vi "BMU参数读取-Auto.vi"(7 "Socket":dbl, 8 "CAN端口":u16(ring), 9 "设备索引号":u16(ring), 10 "CAN卡类型":u32(ring)=21, 11 "从板号":u8=1) -> (3 "成功?":bool)   [LabVIEW 2013] (continued)
                  n842 = call <vilib>:"Close Config Data.vi"("error in (no error)"=w1345, "write file if changed (T)"=w1344, "refnum"=w1343) -> ("error out"=w1342:errorcluster, "file path"=w1339:path)  [unwired: 7 in]
                  n843 = call <vilib>:"MD5Checksum File.vi"("error in (no error)"=w1342, "Path"=w1339) -> ("error out"=w1340:errorcluster, "MD5 message-digest"=w1348:string)  [unwired: 8 in]
                  n844 = Equal?(x=w1348, y=w1347) -> (x = y?=w1346:bool)
                  n845 = Delete(path (use dialog)=w1339, error in=w1340) -> (error out=w1338:errorcluster)  [unwired: 3 in, 2 out]
                  n846 = call <vilib>:"Clear Errors.vi"("error in (no error)"=w1338) -> ()  [unwired: 6 in, 1 out]
                }
              }
              n847 = global write "配置文件全局.vi" "诊断标定读取地址"(w1318) -> ()
              n848 = And(x=w1319, y=w1320) -> (x .and. y?=w1321:bool)
              n849 = control-ref of="结果"() -> (w1326:refnum<vi>)
              n850 = case shown="真" w1321 {
                tunnel: w1307 -> [_ w1370]
                tunnel: w1326 -> [w1356 w1369]
                tunnel: w1320 -> [w1355 _]
                tunnel: w1319 -> [w1354 _]
                frame False {
                  n851 = stacked-sequence {
                    tunnel: w1354 -> [w1358 _]
                    tunnel: w1356 -> [w1357 w1364]
                    tunnel: w1355 -> [_ w1363]
                    frame #0 {
                      n852 = case shown="假" w1358 {
                        tunnel: w1357 -> [w1360 _]
                        frame False {
                          n853 = Build Array("文件格式错误") -> (w1361:string[])
                          n854 = call "表格编辑.vi"("新元素/子数组"=w1361, "活动单元格:单元格背景色"=u32 16711680, "MCListbox引用句柄"=w1360) -> ()  [unwired: 9 out]
                        }
                        frame True {
                        }
                      }
                    }
                    frame #1 {
                      n855 = case shown="假" w1363 {
                        tunnel: w1364 -> [w1366 _]
                        frame False {
                          n856 = Build Array("文件MD5码验证错误") -> (w1367:string[])
                          n857 = call "表格编辑.vi"("新元素/子数组"=w1367, "活动单元格:单元格背景色"=u32 16711680, "MCListbox引用句柄"=w1366) -> ()  [unwired: 9 out]
                        }
                        frame True {
                        }
                      }
                    }
                  }
                  n858 = call <vilib>:"Unset Busy.vi"() -> ()  [unwired: 11 in, 1 out]
                }
                frame True {
                  n859 = stacked-sequence {
                    seq-local: [w1375 _ _ _] -> [_ w1603 w1697 _]
                    seq-local: [w1373 _ _ _] -> [_ w1581 _ _]
                    tunnel: w1370 -> [w1371 _ _ _]
                    tunnel: w1369 -> [w1388 _ _ w1724]
                    frame #0 {
                      w1372 = string[][] []
                      w1385 = "总信息" ("section")
                      n860 = local write "路径"(w1371) -> ()
                      n861 = call <vilib>:"Open Config Data.vi"("create file if necessary (T)"=FALSE, "configuration file path"=w1371) -> ("error out"=w1376:errorcluster, "refnum"=w1375:T26)  [unwired: 7 in, 1 out]
                      n862 = call <vilib>:"Get Key Names.vi"("section"=w1385, "error in (no error)"=w1376, "refnum"=w1375) -> ("key names"=w1384:string[], "refnum out"=w1386:T26)  [unwired: 5 in, 2 out]
                      n863 = for {
                        tunnel: w1386 -> [w1392]
                        tunnel: w1385 -> [w1391]
                        tunnel: w1384 -> [w1390] mode=indexing
                        tunnel: [w1389] -> w1381 mode=indexing
                        n864 = call-poly <vilib>:"Read Key.vi"("section"=w1391, "key"=w1390, "refnum"=w1392) -> ("value"=w1389:string)  [unwired: 5 in, 3 out]
                      }
                      n865 = Index Array(array=w1381) -> (element #1=w1374:string, element #2=w1379:string)  [unwired: 2 in]
                      n866 = Decimal String To Number(string=w1374) -> (number=w1373:i32)  [unwired: 2 in, 1 out]
                      n867 = Concatenate Strings("正在读取" ("字符串"), w1379, "的配置文件" ("字符串")) -> (w1377:string)
                      n868 = Build Array(w1377) -> (w1382:string[])
                      n869 = call "表格编辑.vi"("新元素/子数组"=w1382, "活动单元格:单元格背景色"=u32 6618880, "MCListbox引用句柄"=w1388) -> ()  [unwired: 9 out]
                      n870 = local write "项目信息"(w1372) -> ()
                      n871 = local write "项目信息 2"(w1372) -> ()
                    }
                    frame #1 {
                      w1563 = 20 ("长度")
                      w1604 = "主板" ("section")
                      n872 = call <vilib>:"Get Key Names.vi"("section"=w1604, "refnum"=w1603) -> ("key names"=w1405:string[], "refnum out"=w1605:T26)  [unwired: 6 in, 2 out]
                      n873 = for {
                        tunnel: w1605 -> [w1617]
                        tunnel: w1604 -> [w1616]
                        tunnel: w1405 -> [w1615] mode=indexing
                        tunnel: [w1614] -> w1404 mode=indexing
                        n874 = call-poly <vilib>:"Read Key.vi"("section"=w1616, "key"=w1615, "refnum"=w1617) -> ("value"=w1614:string)  [unwired: 5 in, 3 out]
                      }
                      n875 = Search 1D Array(1D array=w1405, element="总电压过高一级" ("元素"), start index (0)=0 ("开始索引(0)")) -> (index of element=w1485:i32)
                      n876 = Search 1D Array(1D array=w1405, element="风机开启温度" ("元素"), start index (0)=w1485) -> (index of element=w1476:i32)
                      n877 = Search 1D Array(1D array=w1405, element="电池串联" ("元素"), start index (0)=w1476) -> (index of element=w1474:i32)
                      n878 = Decrement(x=w1485) -> (x-1=w1602:i32)
                      n879 = Array Subset(array=w1405, index=1 ("索引"), length=w1602) -> (w1450:string[])
                      n880 = Array Subset(array=w1404, index=1 ("索引"), length=w1602) -> (w1447:string[])
                      n881 = Delete From Array(array=w1447, length=7 ("长度"), index=0 ("索引")) -> (deleted portion=w1444:string[], array with subset deleted=w1394:string[])
                      n882 = Delete From Array(array=w1450, length=7 ("长度"), index=0 ("索引")) -> (array with subset deleted=w1403:string[])  [unwired: 1 out]
                      n883 = Search 1D Array(1D array=w1405, element="分流器型号" ("元素")) -> (index of element=w1408:i32)  [unwired: 1 in]
                      n884 = Index Array(array=w1404, index=0 ("索引")) -> (element=w1578:string)
                      n885 = Decimal String To Number(string=w1578) -> (number=w1395:i32)  [unwired: 2 in, 1 out]
                      n886 = Search 1D Array(1D array=w1403, element="主板电池节数" ("元素")) -> (index of element=w1569:i32)  [unwired: 1 in]
                      n887 = Search 1D Array(1D array=w1403, element="主板温度起始值" ("元素")) -> (index of element=w1566:i32)  [unwired: 1 in]
                      n888 = Search 1D Array(1D array=w1403, element="第一个保险通道" ("元素")) -> (index of element=w1565:i32)  [unwired: 1 in]
                      n889 = Search 1D Array(1D array=w1403, element="主板温度个数" ("元素")) -> (index of element=w1567:i32)  [unwired: 1 in]
                      n890 = Search 1D Array(1D array=w1403, element="主板电压起始值" ("元素")) -> (index of element=w1568:i32)  [unwired: 1 in]
                      n891 = Search 1D Array(1D array=w1403, element="第1通道电压个数" ("元素")) -> (index of element=w1564:i32)  [unwired: 1 in]
                      n892 = Index Array(array=w1404, index=w1408) -> (element=w1407:string)
                      n893 = for {
                        N: 4 -> [_]
                        tunnel: w1444 -> [w1613] mode=indexing
                        tunnel: [w1612] -> w1593 mode=indexing
                        n894 = Fract/Exp String To Number(string=w1613) -> (number=w1612:dbl)  [unwired: 3 in, 1 out]
                      }
                      n895 = Increment(x=w1395) -> (x+1=w1577:i32)
                      n896 = Increment(x=w1395) -> (x+1=w1562:i32)
                      n897 = Increment(x=w1395) -> (x+1=w1575:i32)
                      n898 = Increment(x=w1395) -> (x+1=w1576:i32)
                      n899 = global write "读配置文件全局.vi" "从板个数"(w1395) -> ()
                      n900 = local write "从板个数"(w1395) -> ()
                      n901 = Decimal String To Number(string=w1407) -> (number=w1406:i32)  [unwired: 2 in, 1 out]
                      n902 = Index Array(array=w1444, index #1=4 ("索引"), index #2=5 ("索引"), index #3=6 ("索引")) -> (element #1=w1584:string, element #2=w1583:string, element #3=w1582:string)
                      n903 = Index Array(array=w1593) -> (element #1=w1591:dbl, element #2=w1590:dbl, element #3=w1589:dbl, element #4=w1588:dbl)  [unwired: 4 in]
                      n904 = global write "EV05全局变量1.vi" "分流器型号"(w1406) -> ()
                      n905 = Array Subset(array=w1394, index=w1569, length=w1577) -> (w1561:string[])
                      n906 = Array Subset(array=w1394, index=w1568, length=w1576) -> (w1559:string[])
                      n907 = Array Subset(array=w1394, index=w1567, length=w1575) -> (w1558:string[])
                      n908 = Array Subset(array=w1394, index=w1566, length=w1562) -> (w1557:string[])
                      n909 = Array Subset(array=w1394, index=w1565, length=20 ("长度")) -> (w1556:string[])
                      n910 = Array Subset(array=w1394, index=w1564, length=w1563) -> (w1560:string[])
                      n911 = Multiply(x=w1395, y=2) -> (x*y=w1396:i32)
                      n912 = control-ref of="项目信息2"() -> (w1596:refnum<vi>)
                      n913 = Array Subset(array=w1394, index=0 ("索引"), length=w1396) -> (w1393:string[])
                      n914 = Insert Into Array(array=w1561, new element #1=w1560, new element #2=w1559, new element #3=w1558, new element #4=w1557, new element #5=w1556) -> ()  [unwired: 1 in, 1 out]
                      n915 = property class="Clust (严格)"(reference=w1596) -> (reference out=w1594:refnum<vi>, "Value"=w1595:T10)  [unwired: 1 in, 1 out]
                      n916 = Multiply(x=w1395, y=2) -> (x*y=w1400:i32)
                      n917 = Array Subset(array=w1403, index=w1569, length=w1562) -> (w1434:string[])
                      n918 = Array Subset(array=w1403, index=w1568, length=w1562) -> (w1432:string[])
                      n919 = Array Subset(array=w1403, index=w1567, length=w1562) -> (w1431:string[])
                      n920 = Array Subset(array=w1403, index=w1566) -> (w1430:string[])  [unwired: 1 in]
                      n921 = Array Subset(array=w1403, index=w1565, length=w1563) -> (w1429:string[])
                      n922 = Array Subset(array=w1403, index=w1564, length=w1563) -> (w1433:string[])
                      n923 = Array Subset(array=w1403, index=0 ("索引"), length=w1400) -> (w1399:string[])
                      n924 = global write "读配置文件全局.vi" "表格输入"(w1393) -> ()
                      n925 = Build Array(w1399, w1393) -> (w1555:string[][])
                      n926 = Bundle(cluster=w1595, "电池额定容量(A)"=w1591, "使用者"=w1581, "电池实际容量(A)"=w1590, "车架(牌)号"=w1583, "配置文件版本"=w1582, "SOH(%)"=w1588, "SOC(%)"=w1589, "产品编号"=w1584) -> (w1421:T10)  [unwired: 1 in]
                      n927 = Transpose 2D Array(2D array=w1555) -> (transposed array=w1422:string[][])
                      n928 = Multiply(x=w1395, y=4) -> (x*y=w1426:i32)
                      n929 = Insert Into Array(array=w1434, new element #1=w1433, new element #2=w1432, new element #3=w1431, new element #4=w1430, new element #5=w1429) -> (w1428:string[])  [unwired: 1 in]
                      n930 = Add(x=w1426, y=44) -> (x+y=w1424:i32)
                      n931 = local write "项目信息"(w1422) -> ()
                      n932 = property class="Clust (严格)"(reference=w1594, "Value"=w1421) -> ()  [unwired: 1 in, 2 out]
                      n933 = global write "读配置文件全局.vi" "项目信息"(w1421) -> ()
                      n934 = Array Subset(array=w1404, index=w1474, length=15 ("长度")) -> (w1412:string[])
                      n935 = Array Subset(array=w1428, index=0 ("索引"), length=w1424) -> ()  [unwired: 1 out]
                      n936 = Array Subset(array=w1404, index=w1476, length=15 ("长度")) -> (w1481:string[])
                      n937 = Delete From Array(array=w1412, length=4 ("长度"), index=6 ("索引")) -> (deleted portion=w1468:string[], array with subset deleted=w1467:string[])
                      n938 = for {
                        tunnel: w1481 -> [w1609] mode=indexing
                        tunnel: [w1608] -> w1480 mode=indexing
                        n939 = Fract/Exp String To Number(string=w1609) -> (number=w1608:dbl)  [unwired: 3 in, 1 out]
                      }
                      n940 = for {
                        tunnel: w1467 -> [w1607] mode=indexing
                        tunnel: [w1606] -> w1466 mode=indexing
                        n941 = Fract/Exp String To Number(string=w1607) -> (number=w1606:dbl)  [unwired: 3 in, 1 out]
                      }
                      n942 = Array Subset(array=w1404, index=w1485, length=51 ("长度")) -> (w1554:string[])
                      n943 = for {
                        tunnel: w1554 -> [w1611] mode=indexing
                        tunnel: [w1610] -> w1553 mode=indexing
                        n944 = Fract/Exp String To Number(string=w1611) -> (number=w1610:dbl)  [unwired: 3 in, 1 out]
                      }
                      n945 = Index Array(array=w1466) -> (element #1=w1461:dbl, element #2=w1460:dbl, element #3=w1459:dbl, element #4=w1458:dbl, element #5=w1457:dbl, element #6=w1456:dbl, element #7=w1455:dbl, element #8=w1454:dbl, element #9=w1453:dbl, element #10=w1452:dbl, element #11=w1451:dbl)  [unwired: 11 in]
                      n946 = Delete From Array(array=w1480, length=7 ("长度"), index=0 ("索引")) -> (deleted portion=w1417:dbl[], array with subset deleted=w1478:dbl[])
                      n947 = Delete From Array(array=w1553, length=17 ("长度"), index=0 ("索引")) -> (deleted portion=w1414:dbl[], array with subset deleted=w1550:dbl[])
                      n948 = Array To Cluster(array=w1417) -> (cluster=w1479:T27)
                      n949 = global write "读配置文件全局.vi" "加热控制参数"(w1417) -> ()
                      n950 = Index Array(array=w1478) -> (element #1=w1442:dbl, element #2=w1441:dbl, element #3=w1440:dbl, element #4=w1439:dbl, element #5=w1438:dbl, element #6=w1437:dbl, element #7=w1436:dbl, element #8=w1435:dbl)  [unwired: 8 in]
                      n951 = Delete From Array(array=w1550, length=17 ("长度"), index=0 ("索引")) -> (deleted portion=w1413:dbl[], array with subset deleted=w1410:dbl[])
                      n952 = Index Array(array=w1468) -> (element #1=w1465:string, element #2=w1464:string, element #3=w1462:string, element #4=w1463:string)  [unwired: 4 in]
                      n953 = local write "加热控制参数"(w1479) -> ()
                      n954 = global write "读配置文件全局.vi" "一级故障"(w1414) -> ()
                      n955 = local read "一级故障 5"() -> (w1443:T13)
                      n956 = control-ref of="电池信息"() -> (w1472:refnum<vi>)
                      n957 = global write "读配置文件全局.vi" "二级故障"(w1413) -> ()
                      n958 = global write "读配置文件全局.vi" "三级故障"(w1410) -> ()
                      n959 = Bundle(cluster=w1443, "最大允许单体电压"=w1442, "最大允许总电压"=w1438, "最小允许单体电压"=w1441, "最大允许充电电流"=w1440, "最小允许充电电流"=w1439, "最大允许充电温度"=w1437, "最小允许充电温度"=w1436, "电流步长"=w1435) -> (w1416:T13)
                      n960 = property class="Clust (严格)"(reference=w1472) -> (reference out=w1473:refnum<vi>, "Value"=w1471:T14)  [unwired: 1 in, 1 out]
                      n961 = Bundle(cluster=w1471, "电池串联"=w1461, "电池并联"=w1460, "累计放电总安时"=w1454, "电池包额定容量"=w1459, "电池包额定能量(kWh)"=w1458, "电池包额定总电压"=w1457, "累计充电总安时"=w1455, "电池充满次数"=w1452, "电池放空次数"=w1453, "电池充电次数"=w1451, "电池生产日期"=w1462, "电池厂家"=w1465, "电池类型"=w1464, "电池包组号"=w1463, "实际容量"=w1456) -> (w1411:T14)  [unwired: 2 in]
                      n962 = Cluster To Array(cluster=w1416) -> (array=w1415:dbl[])
                      n963 = local write "一级故障 5"(w1416) -> ()
                      n964 = global write "读配置文件全局.vi" "充电控制参数"(w1415) -> ()
                      n965 = Index Array(array=w1414) -> (element #1=w1543:dbl, element #2=w1542:dbl, element #3=w1541:dbl, element #4=w1540:dbl, element #5=w1539:dbl, element #6=w1538:dbl, element #7=w1537:dbl, element #8=w1536:dbl, element #9=w1535:dbl, element #10=w1534:dbl, element #11=w1533:dbl, element #12=w1532:dbl, element #13=w1531:dbl, element #14=w1530:dbl, element #15=w1529:dbl, element #16=w1528:dbl, element #17=w1527:dbl)  [unwired: 17 in]
                      n966 = global write "读配置文件全局.vi" "电池信息"(w1411) -> ()
                      n967 = Index Array(array=w1413) -> (element #1=w1510:dbl, element #2=w1511:dbl, element #3=w1512:dbl, element #4=w1513:dbl, element #5=w1514:dbl, element #6=w1515:dbl, element #7=w1516:dbl, element #8=w1517:dbl, element #9=w1518:dbl, element #10=w1519:dbl, element #11=w1520:dbl, element #12=w1521:dbl, element #13=w1522:dbl, element #14=w1523:dbl, element #15=w1524:dbl, element #16=w1525:dbl, element #17=w1526:dbl)  [unwired: 17 in]
                      n968 = Index Array(array=w1410) -> (element #1=w1505:dbl, element #2=w1504:dbl, element #3=w1503:dbl, element #4=w1502:dbl, element #5=w1501:dbl, element #6=w1500:dbl, element #7=w1499:dbl, element #8=w1498:dbl, element #9=w1497:dbl, element #10=w1496:dbl, element #11=w1495:dbl, element #12=w1494:dbl, element #13=w1493:dbl, element #14=w1492:dbl, element #15=w1491:dbl, element #16=w1490:dbl, element #17=w1489:dbl)  [unwired: 17 in]
                      n969 = control-ref of="一级故障 3"() -> (w1488:refnum<vi>)
                      n970 = control-ref of="一级故障 2"() -> (w1507:refnum<vi>)
                      n971 = property class="Clust (严格)"(reference=w1507) -> (reference out=w1509:refnum<vi>, "Value"=w1508:T11)  [unwired: 1 in, 1 out]
                      n972 = property class="Clust (严格)"(reference=w1488) -> (reference out=w1487:refnum<vi>, "Value"=w1506:T11)  [unwired: 1 in, 1 out]
                      n973 = property class="Clust (严格)"(reference=w1473, "Value"=w1411) -> ()  [unwired: 1 in, 2 out]
                      n974 = Bundle(cluster=w1508, "总电压过高"=w1510, "整组电压不均衡"=w1514, "SOC过高"=w1522, "单体电压过高"=w1518, "总电压过低"=w1511, "温度过高"=w1512, "温度过低"=w1513, "单组电压不均衡"=w1515, "整组温度不均衡"=w1516, "单组温度不均衡"=w1517, "单体电压过低"=w1519, "充电电流过高"=w1520, "放电电流过高"=w1521, "SOC过低"=w1523, "内阻过大"=w1524, "极柱温度过高"=w1525, "SOH过低"=w1526) -> (w1419:T11)
                      n975 = property class="Clust (严格)"(reference=w1509, "Value"=w1419) -> ()  [unwired: 1 in, 2 out]
                      n976 = Bundle(cluster=w1506, "总电压过高"=w1505, "整组电压不均衡"=w1501, "SOC过高"=w1493, "单体电压过高"=w1497, "总电压过低"=w1504, "温度过高"=w1503, "温度过低"=w1502, "单组电压不均衡"=w1500, "整组温度不均衡"=w1499, "单组温度不均衡"=w1498, "单体电压过低"=w1496, "充电电流过高"=w1495, "放电电流过高"=w1494, "SOC过低"=w1492, "内阻过大"=w1491, "极柱温度过高"=w1490, "SOH过低"=w1489) -> (w1418:T11)
                      n977 = property class="Clust (严格)"(reference=w1487, "Value"=w1418) -> ()  [unwired: 1 in, 2 out]
                      n978 = control-ref of="一级故障"() -> (w1546:refnum<vi>)
                      n979 = property class="Clust (严格)"(reference=w1546) -> (reference out=w1544:refnum<vi>, "Value"=w1545:T11)  [unwired: 1 in, 1 out]
                      n980 = Bundle(cluster=w1545, "总电压过高"=w1543, "整组电压不均衡"=w1539, "SOC过高"=w1531, "单体电压过高"=w1535, "总电压过低"=w1542, "温度过高"=w1541, "温度过低"=w1540, "单组电压不均衡"=w1538, "整组温度不均衡"=w1537, "单组温度不均衡"=w1536, "单体电压过低"=w1534, "充电电流过高"=w1533, "放电电流过高"=w1532, "SOC过低"=w1530, "内阻过大"=w1529, "极柱温度过高"=w1528, "SOH过低"=w1527) -> (w1420:T11)
                      n981 = property class="Clust (严格)"(reference=w1544, "Value"=w1420) -> ()  [unwired: 1 in, 2 out]
                    }
                    frame #2 {
                      w1682 = 1 ("索引")
                      # "均衡计算-电压高阀值1级"
                      n982 = call <vilib>:"Get Section Names.vi"("refnum"=w1697) -> ("section names"=w1698:string[], "refnum out"=w1702:T26)  [unwired: 8 in, 1 out]
                      n983 = local read "从板号"() -> (w1680:u8)
                      n984 = Delete From Array(array=w1698, length=2 ("长度"), index=0 ("索引")) -> (array with subset deleted=w1701:string[])  [unwired: 1 out]
                      n985 = for {
                        tunnel: w1701 -> [w1718] mode=indexing
                        tunnel: w1702 -> [w1719]
                        tunnel: [w1711] -> w1679 mode=indexing
                        tunnel: [w1710] -> w1623
                        n986 = call <vilib>:"Get Key Names.vi"("section"=w1718, "refnum"=w1719) -> ("key names"=w1710:string[], "refnum out"=w1717:T26)  [unwired: 6 in, 2 out]
                        n987 = for {
                          tunnel: w1710 -> [w1723] mode=indexing
                          tunnel: w1718 -> [w1722]
                          tunnel: w1717 -> [w1721]
                          tunnel: [w1720] -> w1711 mode=indexing
                          n988 = call-poly <vilib>:"Read Key.vi"("section"=w1722, "key"=w1723, "refnum"=w1721) -> ("value"=w1720:string)  [unwired: 5 in, 3 out]
                        }
                        n989 = Index Array(array=w1711, index=0 ("索引")) -> (element=w1714:string)
                        n990 = local read "输出数组"() -> (w1715:string[][])
                        n991 = Decimal String To Number(string=w1714) -> (number=w1713:i32)  [unwired: 2 in, 1 out]
                        n992 = Decrement(x=w1713) -> (x-1=w1709:i32)
                        n993 = Replace Array Subset(array=w1715, new element=w1711, index (col)=w1709) -> (w1712:string[][])  [unwired: 1 in]
                        n994 = local write "输出数组"(w1712) -> ()
                      }
                      "key names" <- w1623
                      n995 = Decrement(x=w1680) -> (x-1=w1696:u8)
                      n996 = Index Array(array=w1679, index (row)=w1696) -> (element=w1622:string[])  [unwired: 1 in]
                      n997 = Search 1D Array(1D array=w1623, element="风机开启温度" ("元素")) -> (index of element=w1685:i32)  [unwired: 1 in]
                      n998 = Search 1D Array(1D array=w1623, element="电压过高一级" ("元素"), start index (0)=w1685) -> (index of element=w1648:i32)
                      n999 = Search 1D Array(1D array=w1623, element="均衡计算-电压高阀值1级" ("元素"), start index (0)=w1648) -> (index of element=w1646:i32)
                      n1000 = Array Subset(array=w1622, index=w1646, length=17 ("长度")) -> (w1645:string[])
                      n1001 = Decrement(x=w1685) -> (x-1=w1683:i32)
                      n1002 = Array Subset(array=w1622, index=w1682, length=w1683) -> (w1620:string[])
                      n1003 = Array Subset(array=w1622, index=w1648, length=21 ("长度")) -> (w1694:string[])
                      n1004 = Array Subset(array=w1623, index=w1682, length=w1683) -> (w1659:string[])
                      n1005 = Index Array(array=w1622, index=0 ("索引")) -> (element=w1654:string)
                      n1006 = Array Subset(array=w1622, index=w1685, length=7 ("长度")) -> (w1688:string[])
                      n1007 = for {
                        tunnel: w1645 -> [w1704] mode=indexing
                        tunnel: [w1703] -> w1644 mode=indexing
                        n1008 = Fract/Exp String To Number(string=w1704) -> (number=w1703:dbl)  [unwired: 3 in, 1 out]
                      }
                      n1009 = for {
                        tunnel: w1694 -> [w1706] mode=indexing
                        tunnel: [w1705] -> w1695 mode=indexing
                        n1010 = Fract/Exp String To Number(string=w1706) -> (number=w1705:dbl)  [unwired: 3 in, 1 out]
                      }
                      n1011 = Decimal String To Number(string=w1654) -> (number=w1653:i32)  [unwired: 2 in, 1 out]
                      n1012 = for {
                        tunnel: w1688 -> [w1708] mode=indexing
                        tunnel: [w1707] -> w1656 mode=indexing
                        n1013 = Fract/Exp String To Number(string=w1708) -> (number=w1707:dbl)  [unwired: 3 in, 1 out]
                      }
                      n1014 = global write "读配置文件全局2.vi" "从板板号"(w1653) -> ()
                      n1015 = Delete From Array(array=w1695, length=7 ("长度"), index=0 ("索引")) -> (deleted portion=w1658:dbl[], array with subset deleted=w1691:dbl[])
                      n1016 = Array To Cluster(array=w1656) -> (cluster=w1678:T27)
                      n1017 = Delete From Array(array=w1691, length=7 ("长度"), index=0 ("索引")) -> (deleted portion=w1651:dbl[], array with subset deleted=w1652:dbl[])
                      n1018 = local write "加热控制参数"(w1678) -> ()
                      n1019 = global write "读配置文件全局2.vi" "加热控制参数"(w1656) -> ()
                      n1020 = Array To Cluster(array=w1658) -> (cluster=w1662:T27)
                      n1021 = Array To Cluster(array=w1652) -> (cluster=w1660:T27)
                      n1022 = Array To Cluster(array=w1651) -> (cluster=w1661:T27)
                      n1023 = global write "读配置文件全局2.vi" "三级故障阀值"(w1652) -> ()
                      n1024 = global write "读配置文件全局2.vi" "一级故障阀值"(w1658) -> ()
                      n1025 = global write "读配置文件全局2.vi" "二级故障阀值"(w1651) -> ()
                      n1026 = local write "一级故障 6"(w1662) -> ()
                      n1027 = local write "一级故障 8"(w1660) -> ()
                      n1028 = local write "一级故障 7"(w1661) -> ()
                      n1029 = Search 1D Array(1D array=w1659, element="第1通道电压个数" ("元素")) -> (index of element=w1670:i32)  [unwired: 1 in]
                      n1030 = Search 1D Array(1D array=w1659, element="电压个数" ("元素")) -> ()  [unwired: 1 in, 1 out]
                      n1031 = Search 1D Array(1D array=w1659, element="温度个数" ("元素")) -> (index of element=w1672:i32)  [unwired: 1 in]
                      n1032 = Search 1D Array(1D array=w1659, element="第一个保险通道" ("元素")) -> (index of element=w1671:i32)  [unwired: 1 in]
                      n1033 = Array Subset(array=w1620, length=2 ("长度")) -> (w1667:string[])  [unwired: 1 in]
                      n1034 = Array Subset(array=w1620, index=w1672, length=2 ("长度")) -> (w1665:string[])
                      n1035 = Array Subset(array=w1620, index=w1671, length=20 ("长度")) -> (w1664:string[])
                      n1036 = Array Subset(array=w1620, index=w1670, length=20 ("长度")) -> (w1666:string[])
                      n1037 = Array Subset(array=w1620, length=27 ("长度")) -> (w1619:string[])  [unwired: 1 in]
                      n1038 = Insert Into Array(array=w1667, new element #1=w1666, new element #2=w1665, new element #3=w1664) -> ()  [unwired: 1 in, 1 out]
                      n1039 = Build Array(string[] ["电压个数", "温度个数", "第一个保险通道", "第一个保险位置", "第二个保险通道", "第二个保险位置", "第三个保险通道", "第三个保险位置", "第四个保险通道", "第四个保险位置", "第五个保险通道", "第五个保险位置", "第六个保险通道", "第六个保险位置", "第七个保险通道", "第七个保险位置", "第八个保险通道", "第八个保险位置", "第九个保险通道", "第九个保险位置", "第十个保险通道", "第十个保险位置", "第1通道电压个数", "第2通道电压个数", "第3通道电压个数", "第4通道电压个数", "第5通道电压个数"], w1619) -> (w1663:string[][])
                      n1040 = global write "读配置文件全局2.vi" "表格"(w1619) -> ()
                      n1041 = Index Array(array=w1644) -> (element #1=w1641:dbl, element #2=w1640:dbl, element #3=w1639:dbl, element #4=w1638:dbl, element #5=w1637:dbl, element #6=w1636:dbl, element #7=w1635:dbl, element #8=w1634:dbl, element #9=w1633:dbl, element #10=w1632:dbl, element #11=w1631:dbl, element #12=w1630:dbl, element #13=w1629:dbl, element #14=w1628:dbl, element #15=w1627:dbl, element #16=w1626:dbl, element #17=w1625:dbl, element #18=w1624:dbl)  [unwired: 18 in]
                      n1042 = Transpose 2D Array(2D array=w1663) -> (transposed array=w1657:string[][])
                      n1043 = local write "项目信息 2"(w1657) -> ()
                      n1044 = local read "均衡参数"() -> (w1643:T18)
                      n1045 = Bundle(cluster=w1643, "充电结束电压(90%)"=w1634, "充电结束电压(91%)"=w1633, "充电结束电压(92%)"=w1632, "充电结束电压(93%)"=w1631, "充电结束电压(94%)"=w1630, "均衡计算-电压高阀值1级"=w1641, "均衡计算-电压高阀值2级"=w1640, "均衡计算-电压低阀值1级"=w1639, "均衡计算-电压低阀值2级"=w1638, "均衡计算-最低电压阀值"=w1637, "均衡停止-最低电压阀值"=w1636, "均衡计算-电压极差阀值"=w1635, "充电结束电压(95%)"=w1629, "充电结束电压(96%)"=w1628, "充电结束电压(97%)"=w1627, "充电结束电压(98%)"=w1626, "充电结束电压(99%)"=w1625, "充电结束电压(100%)"=w1624) -> (w1642:T18)
                      n1046 = local write "均衡参数"(w1642) -> ()
                    }
                    frame #3 {
                      n1047 = call <vilib>:"Unset Busy.vi"() -> ()  [unwired: 11 in, 1 out]
                      n1048 = Build Array("读取完成") -> (w1727:string[])
                      n1049 = property on="全部写入" class="Bool (严格)"("DisabledEnum"=0) -> ()  [unwired: 2 in, 2 out]
                      n1050 = call "表格编辑.vi"("新元素/子数组"=w1727, "活动单元格:单元格背景色"=u32 6618880, "MCListbox引用句柄"=w1724) -> ()  [unwired: 9 out]
                    }
                  }
                }
              }
            }
            frame #2 {
              (unwired) "均衡参数"
              # "去掉加热控制信息 20140106"
              n1051 = local read "主从选择"() -> (w1732:enum32{"主板", "从板"})
              n1052 = case shown="\"主板\", 默认" w1732 {
                tunnel: [string[] ["项目信息", "一级故障阀值", "二级故障阀值", "三级故障阀值", "加热控制信息", "充电控制信息", "电池信息", "二维码"] string[] ["从板信息", "一级故障阀值", "二级故障阀值", "三级故障阀值", "二维码"]] -> w1731
                frame "主板", Default {
                }
                frame "从板" {
                }
              }
              n1053 = Array Size(array=w1731) -> (size(s)=w1730:i32)
              n1054 = for {
                tunnel: w1731 -> [w1748] mode=indexing
                tunnel: w1732 -> [w1736]
                tunnel: w1730 -> [w1740]
                tunnel: [w1735] -> w1729
                i -> [w1737]
                n1055 = case shown="\"主板\", 默认" w1736 {
                  tunnel: [w2045 w2076] -> w1742
                  tunnel: [w2044 w2077] -> w1743
                  tunnel: w1748 -> [w2041 w2073]
                  tunnel: [u8 0 ("板号") w2074] -> w1747
                  tunnel: [u8 0 ("板号") u8 0 ("板号")] -> w1746
                  tunnel: [w2040 w2072] -> w1744
                  frame "主板", Default {
                    n1056 = case shown="\"项目信息\"" w2041 {
                      tunnel: [_ u8[] [1, 2, 3, 4, 5, 6, 13, 8, 7, 9, 10, 11, 12] u8[] [1] u8[] [1] u8[] [2] u8[] [3] u8[] [1] u8[] [2] u8[] [1, 2, 3] u8[] [1, 2, 3, 4]] -> w2045
                      tunnel: [_ u8 128 ("命令") u8 140 ("命令") u8 129 ("命令") u8 129 ("命令") u8 129 ("命令") u8 130 ("命令") u8 130 ("命令") u8 131 ("命令") u8 132 ("命令")] -> w2044
                      tunnel: [_ string[] ["产品编号", "电压个数", "通道电压数", "电压起始值", "温度个数", "温度起始值", "保险位置", "电池额定实际容量", "SOC", "配置文件版本", "参数修改记录", "车牌号", "SOH"] string[] ["读二维码"] string[] ["一级故障阀值"] string[] ["二级故障阀值"] string[] ["三级故障阀值"] string[] ["加热控制参数"] string[] ["充电控制参数"] _ string[] ["电池信息1", "电池包组号", "充放电安时", "电池充放电次数"]] -> w2040
                      frame "假", Default {
                      }
                      frame "项目信息" {
                      }
                      frame "二维码" {
                      }
                      frame "一级故障阀值" {
                      }
                      frame "二级故障阀值" {
                      }
                      frame "三级故障阀值" {
                      }
                      frame "加热控制信息" {
                      }
                      frame "充电控制信息" {
                      }
                      frame "历史信息" {
                      }
                      frame "电池信息" {
                      }
                    }
                  }
                  frame "从板" {
                    n1057 = case shown="\"二维码\"" w2073 {
                      tunnel: [_ u8 0 ("命令") u8 10 ("命令") u8 2 ("命令") u8 2 ("命令") u8 2 ("命令") u8 3 ("命令") u8 6 ("命令")] -> w2077
                      tunnel: [_ u8[] [6, 1, 2, 3, 4, 5] u8[] [1] u8[] [1] u8[] [2] u8[] [3] u8[] [1, 2, 3, 4, 5, 6, 7] u8[] [1, 2]] -> w2076
                      tunnel: [_ string[] ["从板号", "电压起始值", "通道电压节数", "保险位置", "温度起始值", "加热控制参数"] string[] ["读二维码"] string[] ["一级故障阀值"] string[] ["二级故障阀值"] string[] ["三级故障阀值"] string[] ["电池包信息1", "电池包序号", "充放电安时", "充电次数时间", "SOC", "车牌号", "充电参数"] string[] ["均衡阀值", "充电结束电压"]] -> w2072
                      frame "假", Default {
                      }
                      frame "从板信息" {
                      }
                      frame "二维码" {
                      }
                      frame "一级故障阀值" {
                      }
                      frame "二级故障阀值" {
                      }
                      frame "三级故障阀值" {
                      }
                      frame "快换参数" {
                      }
                      frame "均衡参数" {
                      }
                    }
                    n1058 = local read "从板号"() -> (w2074:u8)
                  }
                }
                n1059 = Increment(x=w1737) -> (x+1=w1739:i32)
                n1060 = Equal?(x=w1740, y=w1739) -> (x = y?=w1738:bool)
                n1061 = case shown="\"从板\"" w1736 {
                  tunnel: w1737 -> [w2011 w2025]
                  frame "主板", Default {
                    n1062 = case shown="0, 默认" w2011 {
                      tunnel: [T9."项目信息" ("主从板") T9."一级故障阀值" ("主从板") T9."二级故障阀值" ("主从板") T9."三级故障阀值" ("主从板") T9."控制参数" ("主从板") T9."电池信息" ("主从板")] -> w2010
                      frame 0, Default {
                        n1063 = local write "1"(TRUE ("1")) -> ()
                      }
                      frame 1 {
                        n1064 = local write "1 2"(TRUE ("1 2")) -> ()
                      }
                      frame 2 {
                        n1065 = local write "1 3"(TRUE ("1 3")) -> ()
                      }
                      frame 3 {
                        n1066 = local write "1 4"(TRUE ("1 4")) -> ()
                      }
                      frame 4, 5 {
                        n1067 = local write "1 5"(TRUE ("1 5")) -> ()
                      }
                      frame 6 {
                        n1068 = local write "1 11"(TRUE ("1 11")) -> ()
                      }
                    }
                    n1069 = local write "主板2"(w2010) -> ()
                  }
                  frame "从板" {
                    n1070 = case shown="4" w2025 {
                      tunnel: [T20."从板信息" ("等级 2") T20."从板信息" ("等级 2") T20."一级故障阀值" ("等级 2") T20."二级故障阀值" ("等级 2") T20."三级故障阀值" ("等级 2") T20."快换参数" ("等级 2") T15."从板信息" ("等级 2")] -> w2024
                      frame 99, Default {
                        n1071 = local write "1 6"(TRUE ("1 6")) -> ()
                      }
                      frame 0 {
                        n1072 = local write "1 6"(TRUE ("1 6")) -> ()
                      }
                      frame 1 {
                        n1073 = local write "1 7"(TRUE ("1 7")) -> ()
                      }
                      frame 2 {
                        n1074 = local write "1 8"(TRUE ("1 8")) -> ()
                      }
                      frame 3 {
                        n1075 = local write "1 9"(TRUE ("1 9")) -> ()
                      }
                      frame 5 {
                        n1076 = local write "1 10"(TRUE ("1 10")) -> ()
                      }
                      frame 4 {
                        n1077 = local write "1 12"(TRUE ("1 10")) -> ()
                      }
                    }
                    n1078 = local write "等级 2"(w2024) -> ()
                  }
                }
                n1079 = Array Size(array=w1742) -> (size(s)=w1741:i32)
                n1080 = local write "命令"(w1743) -> ()
                n1081 = Build Array(w1746) -> (w1745:u8[])
                n1082 = while {
                  tunnel: w1743 -> [w1780]
                  tunnel: w1747 -> [w1779]
                  tunnel: w1745 -> [w1778]
                  tunnel: w1741 -> [w1774]
                  tunnel: w1738 -> [w1777]
                  tunnel: w1736 -> [w1771]
                  tunnel: [w1770] -> w1735
                  shift-right: [w1769] -> _
                  shift-left: w1744 -> [w1750]
                  shift-right: [w1760] -> _
                  shift-left: w1742 -> [w1749]
                  i -> [w1775]
                  stop <- w1770 stop-if-true
                  n1083 = local read "强制终止读写标记"() -> (w1766:bool)
                  n1084 = Array Size(array=w1750) -> (size(s)=w1768:i32)
                  n1085 = Increment(x=w1775) -> (x+1=w1776:i32)
                  n1086 = Greater Than 0?(x=w1768) -> (x > 0?=w1767:bool)
                  n1087 = Equal?(x=w1774, y=w1776) -> (x = y?=w1772:bool)
                  n1088 = Not(x=w1766) -> (.not. x?=w1765:bool)
                  n1089 = And(x=w1765, y=w1767) -> (x .and. y?=w1764:bool)
                  n1090 = Delete From Array(array=w1750, length=1 ("长度"), index=0 ("索引")) -> (deleted portion=w1756:string[], array with subset deleted=w1761:string[])
                  n1091 = Index Array(array=w1756, index=0 ("索引")) -> (element=w1754:string)
                  n1092 = Delete From Array(array=w1749, length=1 ("长度"), index=0 ("索引")) -> (deleted portion=w1752:u8[], array with subset deleted=w1757:u8[])
                  n1093 = Index Array(array=w1752, index=0 ("索引")) -> (element=w1751:u8)
                  n1094 = case shown="真" w1764 {
                    tunnel: w1780 -> [_ w1796]
                    tunnel: w1751 -> [_ w1795]
                    tunnel: w1779 -> [_ w1794]
                    tunnel: w1778 -> [_ w1793]
                    tunnel: w1754 -> [_ w1792]
                    tunnel: w1777 -> [_ w1791]
                    tunnel: w1772 -> [_ w1790]
                    tunnel: w1771 -> [_ w1789]
                    tunnel: [string[] [] w1785] -> w1769
                    tunnel: w1761 -> [_ w1788]
                    tunnel: [u8[] [] w1783] -> w1760
                    tunnel: w1757 -> [_ w1787]
                    tunnel: w1750 -> [_ w1786]
                    tunnel: w1749 -> [_ w1784]
                    frame False {
                    }
                    frame True {
                      n1095 = while {
                        tunnel: w1796 -> [w1812]
                        tunnel: w1795 -> [w1811]
                        tunnel: w1794 -> [w1810]
                        tunnel: w1793 -> [w1809]
                        tunnel: w1792 -> [w1807]
                        tunnel: w1791 -> [w1806]
                        tunnel: w1790 -> [w1805]
                        tunnel: w1789 -> [w1804]
                        tunnel: w1788 -> [w1800]
                        tunnel: w1787 -> [w1798]
                        tunnel: w1786 -> [w1801]
                        tunnel: [w1802] -> w1785
                        tunnel: w1784 -> [w1799]
                        tunnel: [w1797] -> w1783
                        i -> [w1803]
                        stop <- w1808 stop-if-true
                        n1096 = stacked-sequence {
                          seq-local: [_ _ _ _ w1960 _ _] -> [_ _ _ _ _ w1976 _]
                          tunnel: w1812 -> [_ _ _ w1951 _ _ _]
                          tunnel: w1811 -> [_ _ _ w1950 _ _ _]
                          tunnel: w1810 -> [_ _ _ w1949 _ _ _]
                          tunnel: w1809 -> [_ _ _ w1948 _ _ _]
                          tunnel: [_ _ _ _ w1961 _ _] -> w1808
                          tunnel: w1807 -> [w1814 _ _ _ _ w1975 _]
                          tunnel: w1806 -> [_ _ _ _ _ _ w2003]
                          tunnel: w1805 -> [_ _ _ _ _ _ w2001]
                          tunnel: w1804 -> [w1813 _ _ _ _ _ _]
                          tunnel: w1803 -> [_ _ _ _ _ _ _]
                          tunnel: [_ _ _ _ _ w1974 _] -> w1802
                          tunnel: w1801 -> [_ _ _ _ _ w1973 _]
                          tunnel: w1800 -> [_ _ _ _ _ w1972 _]
                          tunnel: w1799 -> [_ _ _ _ _ w1971 _]
                          tunnel: w1798 -> [_ _ _ _ _ w1970 _]
                          tunnel: [_ _ _ _ _ w1969 _] -> w1797
                          frame #0 {
                            n1097 = case shown="\"从板\"" w1813 {
                              tunnel: w1814 -> [w1815 w1906]
                              frame "主板", Default {
                                n1098 = case shown="\"电压个数\"" w1815 {
                                frame "假", Default {
                                }
                                frame "产品编号" {
                                n1099 = control-ref of="产品编号"() -> (w1817:refnum<vi>)
                                n1100 = property class="Str"(reference=w1817, "Value"="") -> ()  [unwired: 1 in, 2 out]
                                }
                                frame "电压个数" {
                                n1101 = local read "从板个数"() -> (w1818:dbl)
                                n1102 = control-ref of="项目信息"() -> (w1822:refnum<vi>)
                                n1103 = for {
                                N: w1818 -> [_]
                                tunnel: [""] -> w1821 mode=indexing
                                }
                                n1104 = call "表格数据输入-8.6.vi"("行数"=u32 0, "列数"=u32 1, "字符串数组"=w1821, "表格引用"=w1822) -> ()  [unwired: 8 in]
                                }
                                frame "通道电压数" {
                                n1105 = disable-structure shown="禁用" {
                                frame Disabled {
                                n1106 = control-ref of="项目信息"() -> (w1828:refnum<vi>)
                                n1107 = for {
                                N: 20 -> [_]
                                tunnel: [""] -> w1827 mode=indexing
                                }
                                n1108 = local read "从板个数"() -> (w1829:dbl)
                                n1109 = Increment(x=w1829) -> (x+1=w1825:dbl)
                                n1110 = call "表格数据输入-8.6.vi"("行数"=w1825, "列数"=u32 1, "字符串数组"=w1827, "表格引用"=w1828) -> ()  [unwired: 8 in]
                                }
                                frame Enabled {
                                }
                                }
                                }
                                frame "电压起始值" {
                                n1111 = disable-structure shown="禁用" {
                                frame Disabled {
                                n1112 = local read "从板个数"() -> (w1833:dbl)
                                n1113 = Increment(x=w1833) -> (x+1=w1832:dbl)
                                n1114 = control-ref of="项目信息"() -> (w1839:refnum<vi>)
                                n1115 = for {
                                N: w1832 -> [_]
                                tunnel: [""] -> w1838 mode=indexing
                                }
                                n1116 = Multiply(x=u8 1, y=w1833) -> (x*y=w1835:dbl)
                                n1117 = Add(x=w1835, y=u8 21) -> (x+y=w1831:dbl)
                                n1118 = call "表格数据输入-8.6.vi"("行数"=w1831, "列数"=u32 1, "字符串数组"=w1838, "表格引用"=w1839) -> ()  [unwired: 8 in]
                                }
                                frame Enabled {
                                }
                                }
                                }
                                frame "温度个数" {
                                n1119 = local read "从板个数"() -> (w1843:dbl)
                                n1120 = Increment(x=w1843) -> (x+1=w1842:dbl)
                                n1121 = control-ref of="项目信息"() -> (w1849:refnum<vi>)
                                n1122 = for {
                                N: w1842 -> [_]
                                tunnel: [""] -> w1848 mode=indexing
                                }
                                n1123 = Multiply(x=u8 2, y=w1843) -> (x*y=w1845:dbl)
                                n1124 = Add(x=w1845, y=u8 22) -> (x+y=w1841:dbl)
                                n1125 = call "表格数据输入-8.6.vi"("行数"=w1841, "列数"=u32 1, "字符串数组"=w1848, "表格引用"=w1849) -> ()  [unwired: 8 in]
                                }
                                frame "温度起始值" {
                                n1126 = disable-structure shown="禁用" {
                                frame Disabled {
                                n1127 = local read "从板个数"() -> (w1853:dbl)
                                n1128 = Increment(x=w1853) -> (x+1=w1852:dbl)
                                n1129 = control-ref of="项目信息"() -> (w1859:refnum<vi>)
                                n1130 = for {
                                N: w1852 -> [_]
                                tunnel: [""] -> w1858 mode=indexing
                                }
                                n1131 = Multiply(x=u8 3, y=w1853) -> (x*y=w1855:dbl)
                                n1132 = Add(x=w1855, y=u8 23) -> (x+y=w1851:dbl)
                                n1133 = call "表格数据输入-8.6.vi"("行数"=w1851, "列数"=u32 1, "字符串数组"=w1858, "表格引用"=w1859) -> ()  [unwired: 8 in]
                                }
                                frame Enabled {
                                }
                                }
                                }
                                frame "保险位置" {
                                n1134 = local read "从板个数"() -> (w1863:dbl)
                                n1135 = control-ref of="项目信息"() -> (w1869:refnum<vi>)
                                n1136 = for {
                                N: 10 -> [_]
                                tunnel: [""] -> w1868 mode=indexing
                                }
                                n1137 = Multiply(x=u8 4, y=w1863) -> (x*y=w1865:dbl)
                                n1138 = Add(x=w1865, y=u8 24) -> (x+y=w1862:dbl)
                                n1139 = call "表格数据输入-8.6.vi"("行数"=w1862, "列数"=u32 1, "字符串数组"=w1868, "表格引用"=w1869) -> ()  [unwired: 8 in]
                                }
                                frame "电池额定实际容量" {
                                w1871 = 0.0 ("值")
                                n1140 = control-ref of="电池实际容量(A)"() -> (w1872:refnum<vi>)
                                n1141 = control-ref of="电池额定容量(A)"() -> (w1873:refnum<vi>)
                                n1142 = property class="DigNum (严格)"(reference=w1872, "Value"=w1871) -> ()  [unwired: 1 in, 2 out]
                                n1143 = property class="DigNum (严格)"(reference=w1873, "Value"=w1871) -> ()  [unwired: 1 in, 2 out]
                                }
                                frame "SOC" {
                                n1144 = control-ref of="SOC(%)"() -> (w1874:refnum<vi>)
                                n1145 = property class="DigNum (严格)"(reference=w1874, "Value"=0.0 ("值")) -> ()  [unwired: 1 in, 2 out]
                                }
                                frame "配置文件版本" {
                                n1146 = control-ref of="配置文件版本"() -> (w1876:refnum<vi>)
                                n1147 = property class="Str"(reference=w1876, "Value"="" ("值")) -> ()  [unwired: 1 in, 2 out]
                                }
                                frame "参数修改记录" {
                                n1148 = control-ref of="使用者"() -> (w1879:refnum<vi>)
                                n1149 = control-ref of="系统时钟"() -> (w1880:refnum<vi>)
                                n1150 = property class="DigNum (严格)"(reference=w1879, "Value"=0.0 ("值")) -> ()  [unwired: 1 in, 2 out]
                                n1151 = property class="Str"(reference=w1880, "Value"="" ("值")) -> ()  [unwired: 1 in, 2 out]
                                }
                                frame "校正时钟" {
                                n1152 = control-ref of="系统时钟"() -> (w1882:refnum<vi>)
                                n1153 = property class="Str"(reference=w1882, "Value"="" ("值")) -> ()  [unwired: 1 in, 2 out]
                                }
                                frame "车牌号" {
                                n1154 = control-ref of="车架(牌)号"() -> (w1884:refnum<vi>)
                                n1155 = property class="Str"(reference=w1884, "Value"="" ("值")) -> ()  [unwired: 1 in, 2 out]
                                }
                                frame "SOH" {
                                n1156 = control-ref of="SOH(%)"() -> (w1887:refnum<vi>)
                                n1157 = property class="DigNum (严格)"(reference=w1887, "Value"=0.0 ("值")) -> ()  [unwired: 1 in, 2 out]
                                }
                                frame "一级故障阀值" {
                                n1158 = local write "一级故障"(T11 {"总电压过高"=0.0, "整组电压不均衡"=0.0, "SOC过高"=0.0, "单体电压过高"=0.0, "总电压过低"=0.0, "温度过高"=0.0, "温度过低"=0.0, "单组电压不均衡"=0.0, "整组温度不均衡"=0.0, "单组温度不均衡"=0.0, "单体电压过低"=0.0, "充电电流过高"=0.0, "放电电流过高"=0.0, "SOC过低"=0.0, "内阻过大"=0.0, "极柱温度过高"=0.0, "SOH过低"=0.0} ("一级故障")) -> ()
                                }
                                frame "二级故障阀值" {
                                n1159 = local write "一级故障 2"(T11 {"总电压过高"=0.0, "整组电压不均衡"=0.0, "SOC过高"=0.0, "单体电压过高"=0.0, "总电压过低"=0.0, "温度过高"=0.0, "温度过低"=0.0, "单组电压不均衡"=0.0, "整组温度不均衡"=0.0, "单组温度不均衡"=0.0, "单体电压过低"=0.0, "充电电流过高"=0.0, "放电电流过高"=0.0, "SOC过低"=0.0, "内阻过大"=0.0, "极柱温度过高"=0.0, "SOH过低"=0.0} ("一级故障")) -> ()
                                }
                                frame "三级故障阀值" {
                                n1160 = local write "一级故障 3"(T11 {"总电压过高"=0.0, "整组电压不均衡"=0.0, "SOC过高"=0.0, "单体电压过高"=0.0, "总电压过低"=0.0, "温度过高"=0.0, "温度过低"=0.0, "单组电压不均衡"=0.0, "整组温度不均衡"=0.0, "单组温度不均衡"=0.0, "单体电压过低"=0.0, "充电电流过高"=0.0, "放电电流过高"=0.0, "SOC过低"=0.0, "内阻过大"=0.0, "极柱温度过高"=0.0, "SOH过低"=0.0} ("一级故障")) -> ()
                                }
                                frame "加热控制参数" {
                                n1161 = local write "加热控制参数"(T12 {"风机开启温度"=0.0, "风机关闭温度"=0.0, "加热开启温度"=0.0, "加热关闭温度"=0.0, "风机开启温差"=0.0, "风机关闭温差"=0.0, "加热关闭温差"=0.0} ("加热控制参数")) -> ()
                                }
                                frame "充电控制参数" {
                                n1162 = local write "一级故障 5"(T13 {"最大允许单体电压"=0.0, "最大允许总电压"=0.0, "最小允许单体电压"=0.0, "最大允许充电电流"=0.0, "最小允许充电电流"=0.0, "最大允许充电温度"=0.0, "最小允许充电温度"=0.0, "电流步长"=0.0} ("一级故障 5")) -> ()
                                }
                                frame "电池信息1" {
                                w1893 = ""
                                w1894 = 0.0 ("电池串联")
                                n1163 = local read "电池信息"() -> (w1896:T14)
                                n1164 = Bundle By Name(cluster=w1896, "电池串联"=w1894, "电池并联"=w1894, "电池包额定容量"=w1894, "电池包额定能量(kWh)"=w1894, "电池包额定总电压"=w1894, "实际容量"=w1894, "电池厂家"=w1893, "电池类型"=w1893, "电池生产日期"=w1893) -> (w1895:T14)
                                n1165 = local write "电池信息"(w1895) -> ()
                                }
                                frame "电池包组号" {
                                n1166 = local read "电池信息"() -> (w1899:T14)
                                n1167 = Bundle By Name(cluster=w1899, "电池包组号"="") -> (w1898:T14)
                                n1168 = local write "电池信息"(w1898) -> ()
                                }
                                frame "充放电安时" {
                                w1900 = 0.0 ("累计充电总安时")
                                n1169 = local read "电池信息"() -> (w1902:T14)
                                n1170 = Bundle By Name(cluster=w1902, "累计充电总安时"=w1900, "累计放电总安时"=w1900) -> (w1901:T14)
                                n1171 = local write "电池信息"(w1901) -> ()
                                }
                                frame "电池充放电次数" {
                                w1903 = 0.0 ("累计充电总安时")
                                n1172 = local read "电池信息"() -> (w1905:T14)
                                n1173 = Bundle By Name(cluster=w1905, "电池充满次数"=w1903, "电池放空次数"=w1903, "电池充电次数"=w1903) -> (w1904:T14)
                                n1174 = local write "电池信息"(w1904) -> ()
                                }
                                }
                              }
                              frame "从板" {
                                n1175 = case shown="\"电压起始值\"" w1906 {
                                frame "假", Default {
                                }
                                frame "电压起始值" {
                                n1176 = control-ref of="项目信息 2"() -> (w1907:refnum<vi>)
                                n1177 = for {
                                N: 1 -> [_]
                                tunnel: [""] -> w1911 mode=indexing
                                }
                                n1178 = call "表格数据输入-8.6.vi"("行数"=u32 0, "列数"=u32 1, "字符串数组"=w1911, "表格引用"=w1907) -> ()  [unwired: 8 in]
                                }
                                frame "通道电压个数" {
                                n1179 = control-ref of="项目信息 2"() -> (w1913:refnum<vi>)
                                n1180 = for {
                                N: 5 -> [_]
                                tunnel: [""] -> w1917 mode=indexing
                                }
                                n1181 = call "表格数据输入-8.6.vi"("行数"=u32 22, "列数"=u32 1, "字符串数组"=w1917, "表格引用"=w1913) -> ()  [unwired: 8 in]
                                }
                                frame "保险位置" {
                                n1182 = control-ref of="项目信息 2"() -> (w1919:refnum<vi>)
                                n1183 = for {
                                N: 10 -> [_]
                                tunnel: [""] -> w1923 mode=indexing
                                }
                                n1184 = call "表格数据输入-8.6.vi"("行数"=u32 2, "列数"=u32 1, "字符串数组"=w1923, "表格引用"=w1919) -> ()  [unwired: 8 in]
                                }
                                frame "温度起始值" {
                                n1185 = control-ref of="项目信息 2"() -> (w1925:refnum<vi>)
                                n1186 = for {
                                N: 1 -> [_]
                                tunnel: [""] -> w1929 mode=indexing
                                }
                                n1187 = call "表格数据输入-8.6.vi"("行数"=u32 1, "列数"=u32 1, "字符串数组"=w1929, "表格引用"=w1925) -> ()  [unwired: 8 in]
                                }
                                frame "加热控制参数" {
                                n1188 = local write "加热控制参数"(T12 {"风机开启温度"=0.0, "风机关闭温度"=0.0, "加热开启温度"=0.0, "加热关闭温度"=0.0, "风机开启温差"=0.0, "风机关闭温差"=0.0, "加热关闭温差"=0.0} ("加热控制参数")) -> ()
                                }
                                frame "一级故障阀值" {
                                n1189 = local write "一级故障 6"(T16 {"电压过高"=0.0, "电压过低"=0.0, "温度过高"=0.0, "温度过低"=0.0, "电压不均衡(V)"=0.0, "温度不均衡"=0.0, "SOC过低"=0.0} ("一级故障 6")) -> ()
                                }
                                frame "二级故障阀值" {
                                n1190 = local write "一级故障 7"(T16 {"电压过高"=0.0, "电压过低"=0.0, "温度过高"=0.0, "温度过低"=0.0, "电压不均衡(V)"=0.0, "温度不均衡"=0.0, "SOC过低"=0.0} ("一级故障 7")) -> ()
                                }
                                frame "三级故障阀值" {
                                n1191 = local write "一级故障 8"(T16 {"电压过高"=0.0, "电压过低"=0.0, "温度过高"=0.0, "温度过低"=0.0, "电压不均衡(V)"=0.0, "温度不均衡"=0.0, "SOC过低"=0.0} ("一级故障 7")) -> ()
                                }
                                frame "均衡参数" {
